vi "Test.vi"() -> ()   [LabVIEW 2024]
panel:
  in  "stop":bool
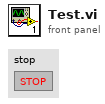
[diagram p1: front panel]
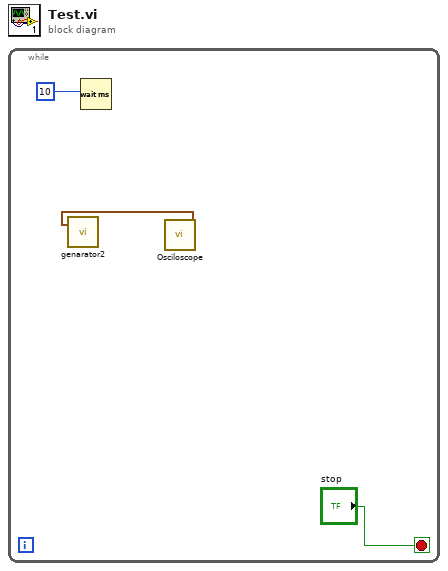
[diagram p0: block diagram]
diagram:
  n1 = while {
    stop <- "stop" stop-if-true
    n2 = call "genarator2.vi"() -> ("Waveform Graph 2"=w1:waveform(dbl))  [unwired: 19 in]
    n3 = Wait (ms)(milliseconds to wait=10) -> ()  [unwired: 1 out]
    n4 = call "Osciloscope.vi"("Waveform Graph"=w1) -> ()  [unwired: 11 in]
  }
